vi "Write Analyze Enq.vi"(8 "error in (no error)":errorcluster, 10 "Actor Framework:Message Enqueuer":refnum<class "Message Enqueuer.lvclass">, 11 "HIJ Vision Display in":refnum<class "HIJ Vision Display.lvclass">) -> (0 "error out":errorcluster, 3 "HIJ Vision Display out":refnum<class "HIJ Vision Display.lvclass">)   [LabVIEW 2014, in "HIJ Vision Display.lvlib" / "HIJ Vision Display.lvclass"]
uses:
  HIJ Vision Display.lvclass
  <vilib>/ActorFramework/Message Enqueuer/Message Enqueuer.lvclass
  HIJ Vision Display.lvclass/HIJ Vision Display.ctl
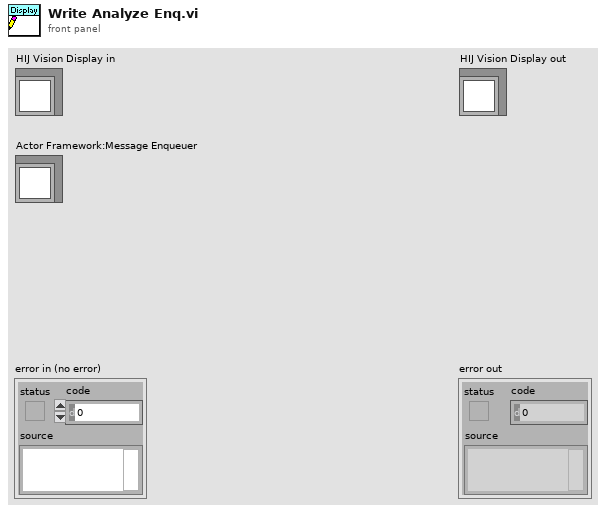
[diagram p1: front panel]
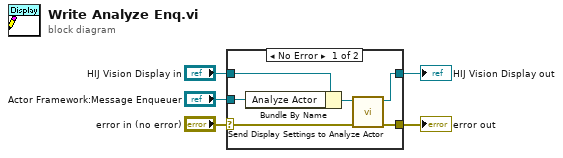
[diagram p0: block diagram]
diagram:
  n1 = case shown="No Error" "error in (no error)" {
    selector: "error in (no error)" -> [w7 w12]
    tunnel: [w6 w12] -> w4
    tunnel: [w8 w13] -> w2
    tunnel: "HIJ Vision Display in" -> [w11 w13]
    tunnel: "Actor Framework:Message Enqueuer" -> [w10 _]
    frame No Error {
      n2 = Bundle By Name(cluster=w11, "Analyze Actor"=w10) -> (w9:refnum<class "HIJ Vision Display.lvclass">)
      n3 = call-dynamic "Send Display Settings to Analyze Actor.vi"("error in (no error)"=w7, "AF IMAQ Display in"=w9) -> ("error out"=w6:errorcluster, "AF IMAQ Display out"=w8:refnum<class "HIJ Vision Display.lvclass">)  [unwired: 8 in]
    }
    frame Error {
    }
  }
  "error out" <- w4
  "HIJ Vision Display out" <- w2
